vi "Get Default Configuration.vi"() -> (2 "Parameters":T1={"Kc"=1.0, "Ti"=0.0, "Td"=0.0, "Min Speed"=0.0, "Max Speed"=100.0})   [LabVIEW 2014, in "Pump.lvclass"]
uses:
  Pump.lvclass
  Parameters - cluster.ctl
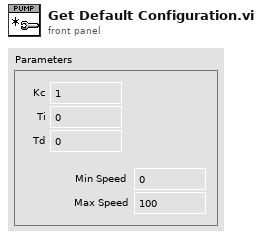
[diagram p1: front panel]
types:
  T1 = typedef "Pump.lvclass/Parameters - cluster.ctl" = cluster{"Kc":dbl, "Ti":dbl, "Td":dbl, "Min Speed":dbl, "Max Speed":dbl}
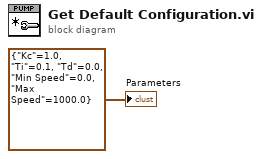
[diagram p0: block diagram]
diagram:
  "Parameters" <- T1 {"Kc"=1.0, "Ti"=0.1, "Td"=0.0, "Min Speed"=0.0, "Max Speed"=1000.0} ("Parameters")
